vi "Create New Files.vi"(8 "error in (no error)":errorcluster, 11 "Base Path":path=path "C:/Users/dgrimm/Desktop/BangBang Raw Data/Written Data") -> (0 "error out":errorcluster, 2 "TDMS File Reference":refnum<k34>, 3 "Binary File Reference":refnum<file>)   [LabVIEW 2021]
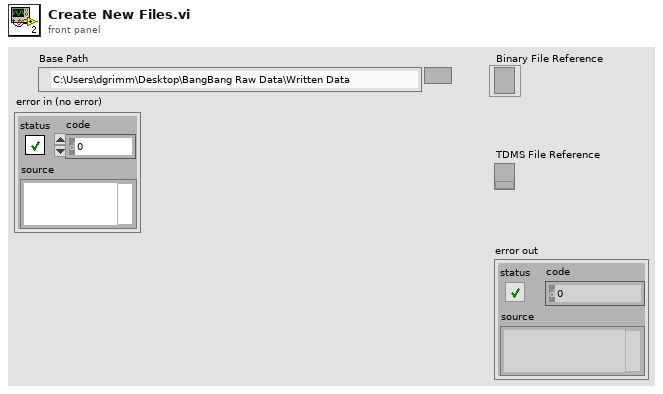
[diagram p1: front panel]
types:
  T1 = enum16{"open", "open or create", "create or replace", "create", "open (read-only)"}
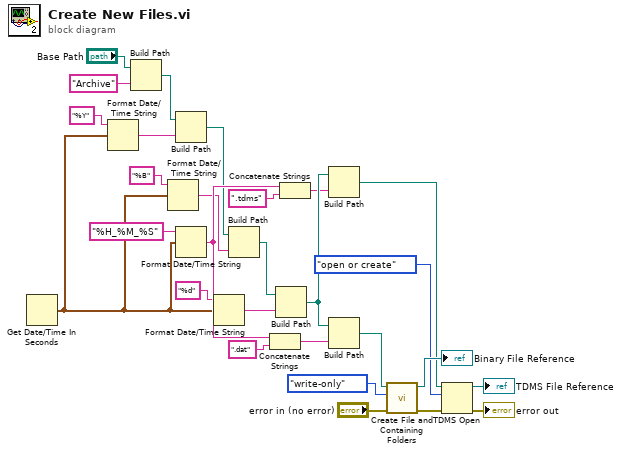
[diagram p0: block diagram]
diagram:
  n1 = Get Date/Time In Seconds() -> (seconds since 1Jan1904=w15:timestamp)
  n2 = Format Date/Time String(time format string (%c)="%Y", seconds (now)=w15) -> (date/time string=w11:string)  [unwired: 1 in]
  n3 = Build Path(base path="Base Path", name or relative path="Archive" ("Folder Name")) -> (appended path=w4:path)
  n4 = Format Date/Time String(time format string (%c)="%B", seconds (now)=w15) -> (date/time string=w12:string)  [unwired: 1 in]
  n5 = Build Path(base path=w4, name or relative path=w11) -> (appended path=w5:path)
  n6 = Format Date/Time String(time format string (%c)="%H_%M_%S", seconds (now)=w15) -> (date/time string=w22:string)  [unwired: 1 in]
  n7 = Format Date/Time String(time format string (%c)="%d", seconds (now)=w15) -> (date/time string=w13:string)  [unwired: 1 in]
  n8 = Build Path(base path=w5, name or relative path=w12) -> (appended path=w6:path)
  n9 = Concatenate Strings(w22, ".dat" ("string")) -> (w23:string)
  n10 = Build Path(base path=w6, name or relative path=w13) -> (appended path=w20:path)
  n11 = Concatenate Strings(w22, ".tdms" ("string")) -> (w7:string)
  n12 = Build Path(base path=w20, name or relative path=w7) -> (appended path=w17:path)
  n13 = Build Path(base path=w20, name or relative path=w23) -> (appended path=w24:path)
  n14 = call <vilib>:"Create File and Containing Folders.vi"("error in (no error)"="error in (no error)", "access"=enum16{"read/write", "read-only", "write-only"}."write-only", "file path"=w24) -> ("error out"=w26:errorcluster, "refnum out"=→"Binary File Reference":refnum<file>)  [unwired: 7 in]
  n15 = TDMS Open(8:w26, 10:T1."open or create" ("operation (0:open)"), 11:w17) -> (0:→"error out":errorcluster, 3:→"TDMS File Reference":refnum<k34>)  [unwired: 4 in]
